vi "sub_position_fgv.vi"(7 "cmd":enum16{"ini", "add"}(ring), 10 "buf size":i32=16, 11 "data":i16) -> (2 "set pt":i16, 3 "buff":i16[](array[numeric]))   [LabVIEW 2018]
uses:
  <vilib>/Analysis/baseanly.llb/Mean (DBL).vi
  <vilib>/Analysis/NI_AALBase.lvlib
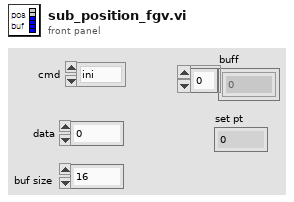
[diagram p1: front panel]
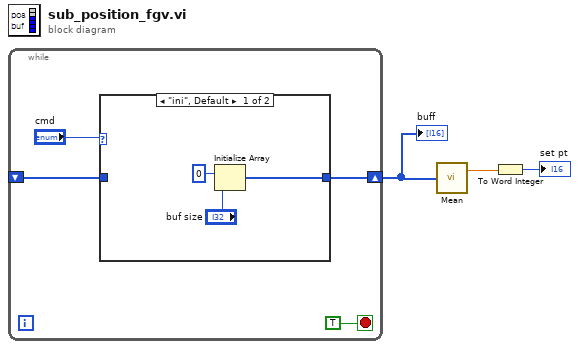
[diagram p0: block diagram]
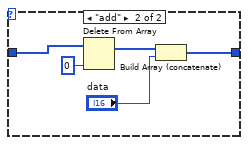
[diagram p2: hidden frame]
diagram:
  n1 = while {
    shift-right: [w5] -> w3
    shift-left: _ -> [w4]
    stop <- TRUE stop-if-true
    n2 = case shown="\"ini\", Default" "cmd" {
      tunnel: [w8 w12] -> w5
      tunnel: w4 -> [_ w13]
      frame "ini", Default {
        n3 = Initialize Array(i16 0 ("element"), "buf size") -> (w8:i16[])
      }
      frame "add" {
        n4 = Delete From Array(array=w13, index=0) -> (array with subset deleted=w15:i16[])  [unwired: 1 in, 1 out]
        n5 = Build Array (concatenate)(w15, "data") -> (w12:i16[])
      }
    }
  }
  "buff" <- w3
  n6 = call-poly <vilib>:"Mean.vi"("X"=w3) -> ("mean"=w2:dbl)  [unwired: 1 out]
  n7 = To Word Integer(number=w2) -> (16bit integer=→"set pt":i16)
